vi "fmt_getUTF-8Text.vi"(8 "error in":errorcluster, 11 "plain text":string) -> (0 "error out":errorcluster, 3 "utf-8 text":string)   [LabVIEW 2017, in "NI_ExcelFile.lvlib"]
uses:
  <vilib>/express/express shared/NI_ExcelFile/NI_ExcelFile.lvlib
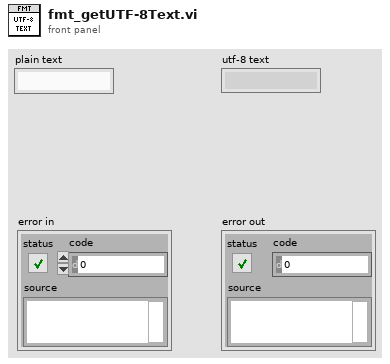
[diagram p1: front panel]
types:
  T1 = enum32{"invalid OS target", "Mac OS", "Windows 3.1", "Windows 95/NT", "Solaris 1", "Solaris 2", "HP-UX", "PowerMAX", "Linux", "Irix", "Rhapsody", "BeOS", "AIX", "OSF1", "VxWorks", "PharLap", "Carbon", "RTX", "Windows x64", "Linux x64", "Mac OS X x64"}
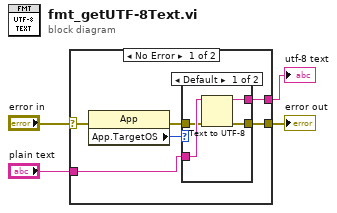
[diagram p0: block diagram]
diagram:
  n1 = case shown="No Error" "error in" {
    selector: "error in" -> [w7 w18]
    tunnel: [w9 w18] -> w4
    tunnel: [w8 w17] -> w3
    tunnel: "plain text" -> [w5 w17]
    frame No Error {
      n2 = property class="App"(error in=w7) -> (error out=w6:errorcluster, "App.TargetOS"=w10:T1)  [unwired: 1 in, 1 out]
      n3 = case shown="Default" w10 {
        tunnel: w5 -> [w14 w16]
        tunnel: w6 -> [w13 w15]
        tunnel: [w12 w15] -> w9
        tunnel: [w11 w16] -> w8
        frame Default {
          n4 = Text to UTF-8(8:w13, 11:w14) -> (0:w12:errorcluster, 3:w11:string)  [unwired: 1 in]
        }
        frame "VxWorks" {
        }
      }
    }
    frame Error {
    }
  }
  "error out" <- w4
  "utf-8 text" <- w3
